vi "syncDAQ_main.vi"() -> ()   [LabVIEW 2013]
uses:
  <vilib>/Utility/error.llb/DialogType.ctl
  <vilib>/DAQmx/read.llb/DAQmx Read (Analog 1D DBL 1Chan NSamp).vi
  <vilib>/DAQmx/read.llb/DAQmx Read (Analog 1D Wfm NChan NSamp).vi
  <vilib>/DAQmx/miscellaneous.llb/DAQmx Fill In Error Info.vi
  <vilib>/ErrorRing/Error Ring.xnode
panel:
  in  "Ratio":dbl=0.3 caption="复位时间比"
  in  "Vx_Max":dbl=3.0 caption="X向最大电压"
  in  "Vy_Max":dbl=3.0 caption="Y向最大电压"
  in  "N_x":i32=512 caption="采样行数"
  in  "N_y":i32=512 caption="每行采样数"
  in  "StopBtn":bool
  in  "每次采集行数":i32=16
  in  "physical channels read":tag="Dev1/ai0" caption="物理通道（读取）"
  in  "physical channels write":tag="Dev1/ao0:1" caption="物理通道（写入）"
  out "number of samples\nper channel":i32=11703 caption="每通道采样数"
  in  "rate":dbl=250000.0 caption="采样速率" format="%#_6f"
  out "data read":waveform(dbl)[](graph) caption="数据输出"
  out "data write":waveform(dbl)[](graph) caption="数据输出"
  in  "采样模式":enum32{"有限采样", "连续采样"}(tab)=enum."连续采样"
  out "Finite Sample Graph":dbl[][](graph)
  out "Continuous sampling graph":dbl[][](graph)
  # "Basic DAQ\nsettings"
  # "Imaging settings"
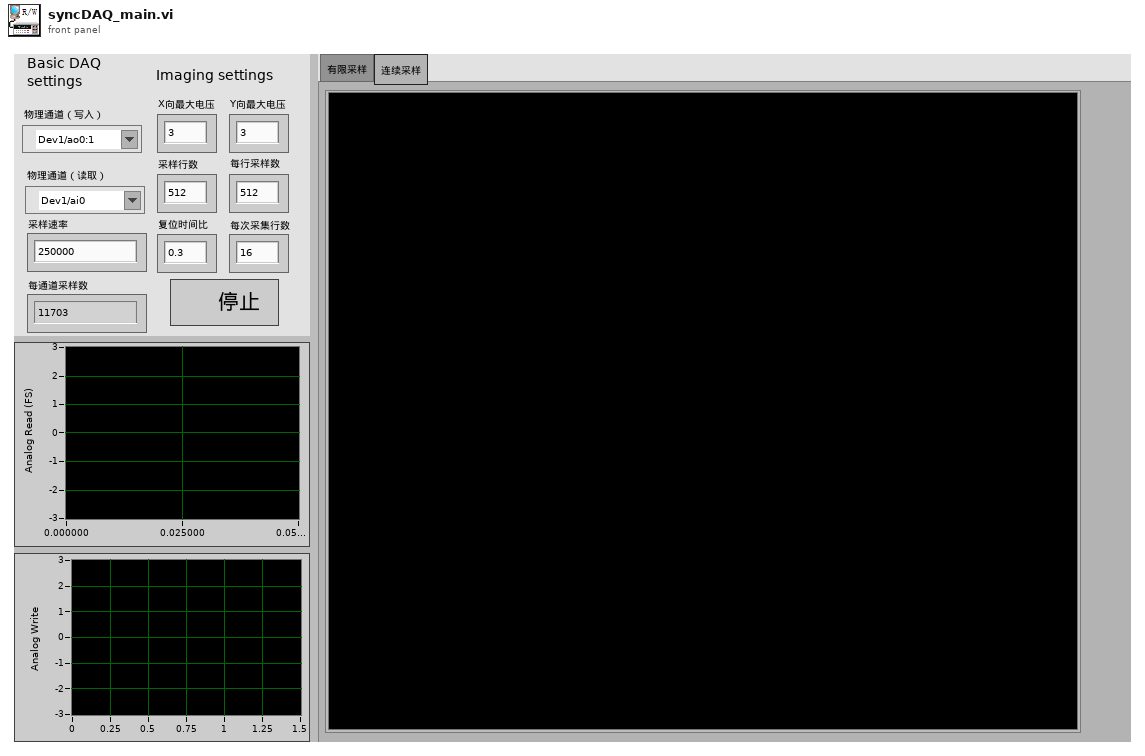
[diagram p1: front panel]
types:
  T1 = enum8{"Enabled", "Disabled", "Disabled and Grayed Out"}
  T2 = cluster{"Vx_Max":dbl, "Vy_Max":dbl, "Tx":dbl, "Row_N":i32, "Ratio":dbl}
  T3 = typedef "DialogType.ctl" = u16
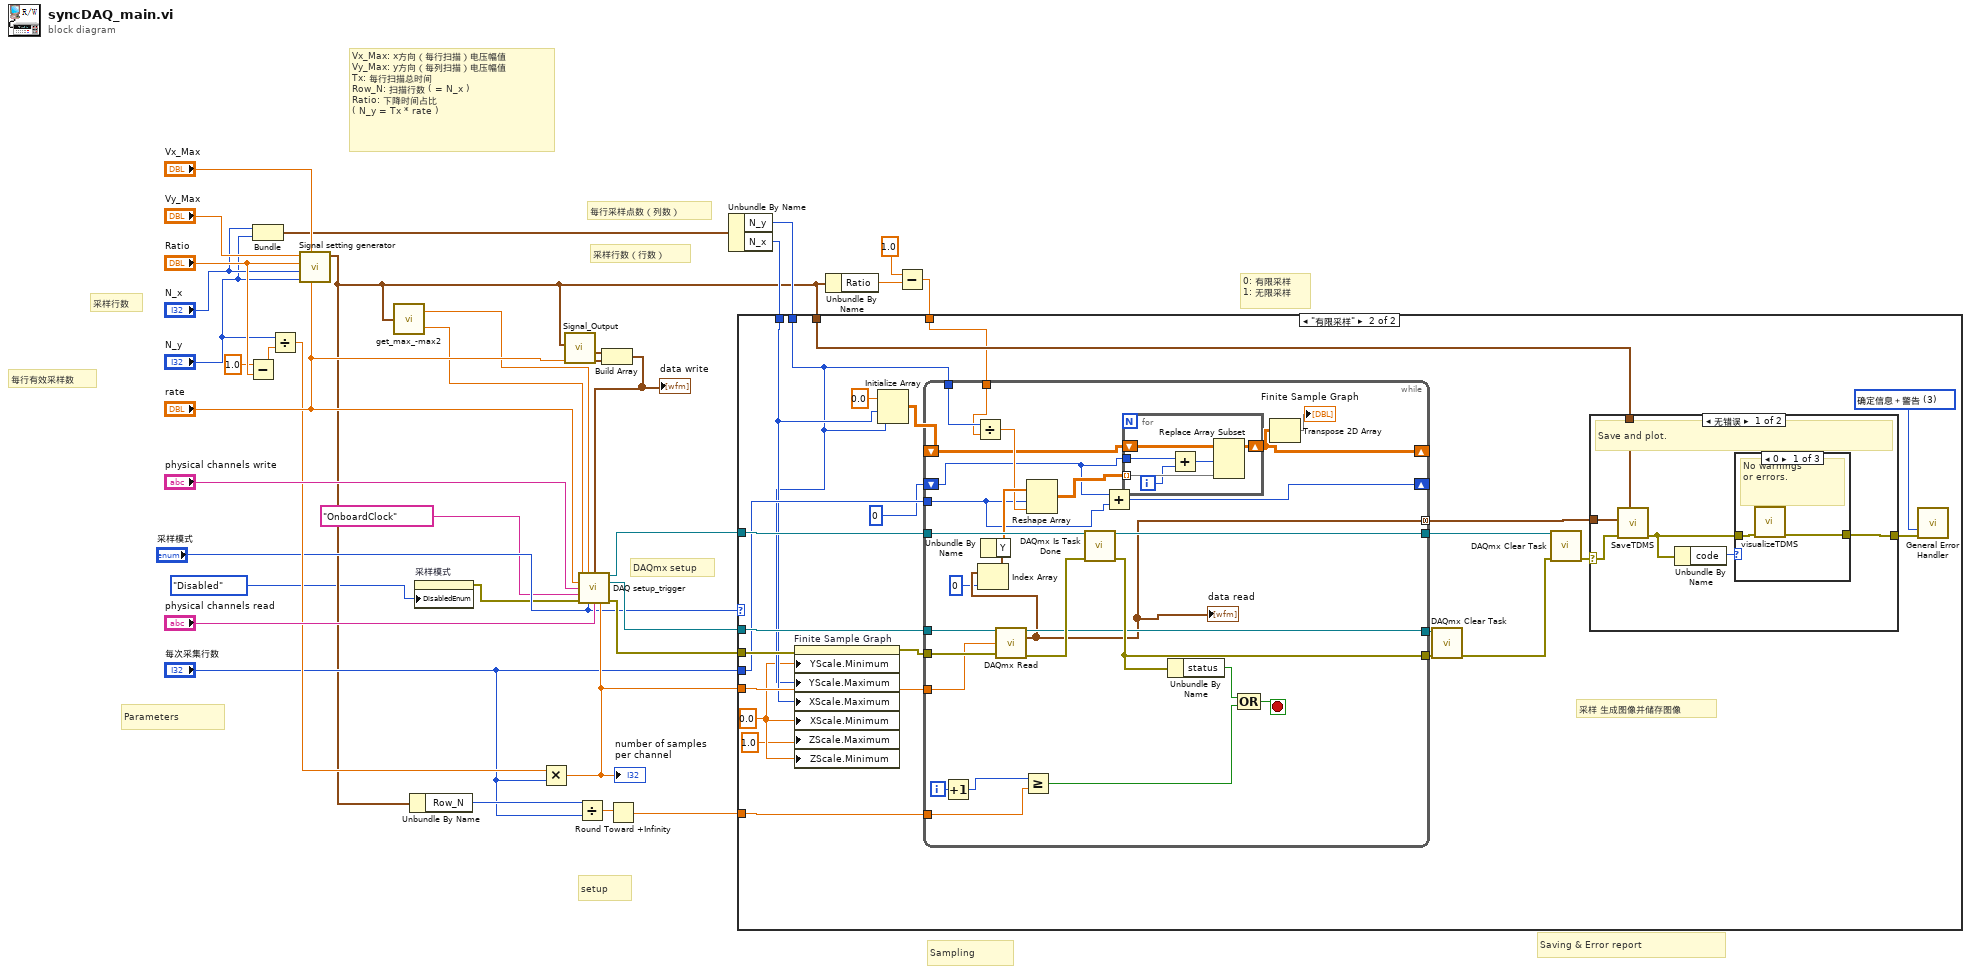
[diagram p0: block diagram]
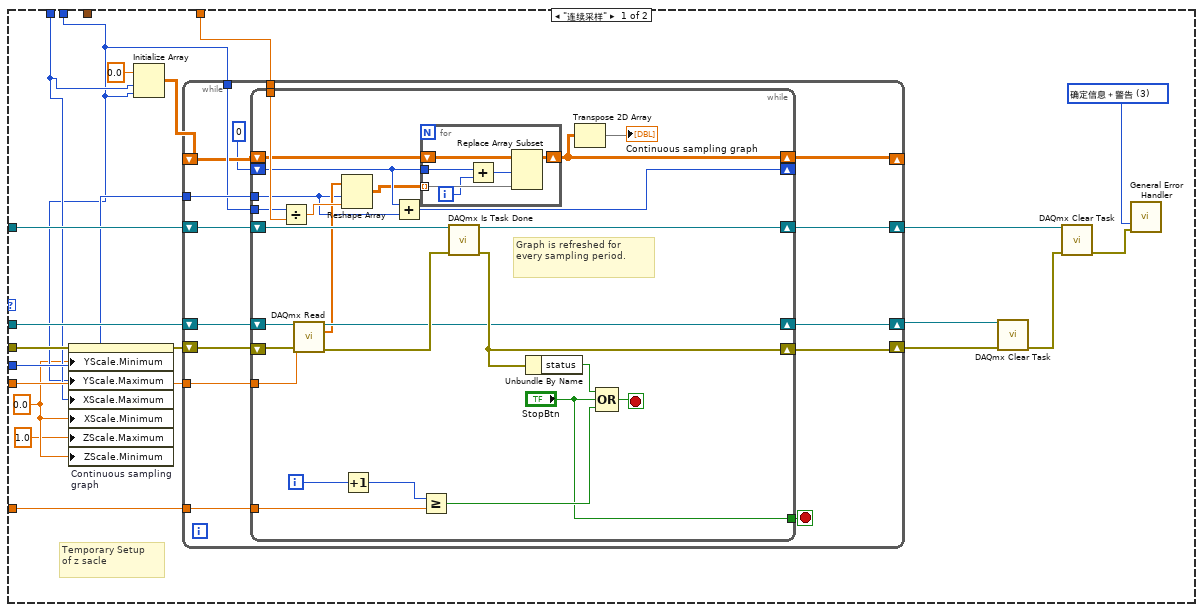
[diagram p2: hidden frame]
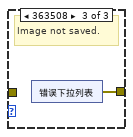
[diagram p4: hidden frame]
diagram:
  # "Vx_Max: x方向（每行扫描）电压幅值\nVy_Max: y方向（每列扫描）电压幅值\nTx: 每行扫描总时间\nRow_N: 扫描行数 ( = N_x )\nRatio: 下降时间占比\n( N_y = Tx * rate )"
  # "采样行数（行数）"
  # "每行采样点数（列数）"
  # "Saving & Error report"
  # "0: 有限采样\n1: 无限采样"
  # "每行有效采样数"
  # "采样行数"
  # "DAQmx setup"
  # "Parameters"
  # "Sampling"
  # "setup"
  n1 = Subtract(x=1.0, y="Ratio") -> (x-y=w22:dbl)
  n2 = Bundle("N_x"="N_x", "N_y"="N_y") -> (w9:cluster{"N_x":i32, "N_y":i32})  [unwired: 1 in]
  n3 = Divide(x="N_y", y=w22) -> (x/y=w21:dbl)
  n4 = call "Signal setting generator.vi"("rate"="rate", "Vx_Max"="Vx_Max", "N_y"="N_y", "N_x"="N_x", "Ratio"="Ratio", "Vy_Max"="Vy_Max") -> ("Waveform out"=w4:T2)  [unwired: 5 in]
  n5 = call "get_max_-max2.vi"("Waveform out"=w4) -> ("-max_xy"=w5:dbl, "max_xy"=w6:dbl)  [unwired: 2 in]
  n6 = Unbundle By Name(w4) -> ("Row_N"=w19:i32)
  n7 = property on="采样模式" class="TabCtl (严格)"("DisabledEnum"=T1."Disabled" ("禁用")) -> (error out=w1:errorcluster)  [unwired: 2 in, 1 out]
  n8 = Multiply(x=w21, y="每次采集行数") -> (x*y=w25:dbl)
  "number of samples\nper channel" <- w25
  n9 = call "Signal_Output.vi"("Fs (Hz)"="rate", "Waveform settings"=w4) -> ("Y"=w29:waveform(dbl), "X"=w30:waveform(dbl))  [unwired: 7 in, 1 out]
  n10 = Divide(x=w19, y="每次采集行数") -> (x/y=w18:dbl)
  n11 = Build Array(w30, w29) -> (w20:waveform(dbl)[])
  "data write" <- w20
  n12 = call "DAQ setup_trigger.vi"("Vx_min"=w5, "Vx_max"=w6, "数组"=w20, "rate"="rate", "physical channels write"="physical channels write", "Timing source"=tag "OnboardClock", "error in"=w1, "sample mode"="采样模式", "physical channels read"="physical channels read", "Number of samples per channel"=w25) -> ("Writing task out"=w35:refnum<k21>, "Reading task out"=w34:refnum<k21>, "错误输出"=w33:errorcluster)  [unwired: 3 in]
  n13 = Round Toward +Infinity(x=w18) -> (ceil(x): smallest int >= x=w17:dbl)
  n14 = Unbundle By Name(w9) -> ("N_y"=w7:i32, "N_x"=w8:i32)
  n15 = Unbundle By Name(w4) -> ("Ratio"=w12:dbl)
  n16 = Subtract(x=1.0, y=w12) -> (x-y=w10:dbl)
  n17 = case shown="\"有限采样\"" "采样模式" {
    tunnel: w35 -> [w55 w126]
    tunnel: w34 -> [w49 w120]
    tunnel: w33 -> [w44 w113]
    tunnel: w25 -> [w48 w117]
    tunnel: w17 -> [w47 w115]
    tunnel: "每次采集行数" -> [w45 w110]
    tunnel: w10 -> [w42 w111]
    tunnel: w8 -> [w40 w106]
    tunnel: w7 -> [w39 w105]
    tunnel: w4 -> [_ w114]
    frame "连续采样" {
      w37 = 0.0 ("X标尺.范围:最小值")
      w50 = T3 3 items=["无对话框", "确定信息", "继续或停止信息", "确定信息＋警告", "继续/停止+警告"] ("type of dialog (OK msg:1)")
      # "Temporary Setup\nof z sacle"
      n18 = property on="Continuous sampling graph" class="IntGraph (严格)"(error in=w44, "YScale.Minimum"=w37, "YScale.Maximum"=w39, "XScale.Maximum"=w40, "XScale.Minimum"=w37, "ZScale.Maximum"=1.0 ("X标尺.范围:最小值"), "ZScale.Minimum"=w37) -> (error out=w43:errorcluster)  [unwired: 1 in, 1 out]
      n19 = Initialize Array(0.0 ("元素"), w40, w39) -> (w38:dbl[][])
      n20 = while {
        tunnel: w48 -> [w66]
        tunnel: w47 -> [w65]
        tunnel: w45 -> [w63]
        tunnel: w42 -> [w62]
        shift-right: [w61] -> w52
        shift-left: w55 -> [w70]
        shift-right: [w69] -> w54
        shift-left: w49 -> [w68]
        shift-right: [w59] -> w53
        shift-left: w43 -> [w67]
        tunnel: w39 -> [w60]
        shift-right: [w57] -> _
        shift-left: w38 -> [w58]
        stop <- w64 stop-if-true
        n21 = while {
          tunnel: w66 -> [w91]
          tunnel: w65 -> [w88]
          shift-right: [w73] -> w57
          shift-left: w58 -> [w74]
          tunnel: ["StopBtn"] -> w64
          tunnel: w63 -> [w75]
          tunnel: w62 -> [w82]
          shift-right: [w81] -> w61
          shift-left: w70 -> [w84]
          shift-right: [w94] -> w69
          shift-left: w68 -> [w92]
          shift-right: [w95] -> w59
          shift-left: w67 -> [w93]
          tunnel: w60 -> [w79]
          shift-right: [w76] -> _
          shift-left: 0 -> [w72]
          i -> [w83]
          stop <- w86 stop-if-true
          # "Graph is refreshed for\nevery sampling period."
          n22 = Divide(x=w79, y=w82) -> (x/y=w80:dbl)
          n23 = call-poly <vilib>:"DAQmx Read.vi"("task/channels in"=w92, "number of samples per channel"=w91, "error in"=w93) -> ("task out"=w94:refnum<k21>, "data"=w77:dbl[], "error out"=w96:errorcluster)  [unwired: 10 in]
          n24 = Reshape Array(w77, w75, w80) -> (w71:dbl[][])
          n25 = Increment(x=w83) -> (x+1=w89:i32)
          n26 = Add(x=w72, y=w75) -> (x+y=w76:i32)
          n27 = for {
            tunnel: w72 -> [w99]
            tunnel: w71 -> [w100] mode=indexing
            shift-right: [w101] -> w73
            shift-left: w74 -> [w102]
            i -> [w98]
            n28 = Add(x=w99, y=w98) -> (x+y=w97:i32)
            n29 = Replace Array Subset(array=w102, new element=w100, index (row)=w97) -> (w101:dbl[][])  [unwired: 1 in]
          }
          n30 = Greater Or Equal?(x=w89, y=w88) -> (x >= y?=w87:bool)
          n31 = call <vilib>:"DAQmx Is Task Done.vi"("task/channels in"=w84, "error in"=w96) -> ("task out"=w81:refnum<k21>, "error out"=w95:errorcluster)  [unwired: 11 in, 1 out]
          n32 = Unbundle By Name(w95) -> ("status"=w90:bool)
          n33 = Transpose 2D Array(2D array=w73) -> (transposed array=→"Continuous sampling graph":dbl[][])
          n34 = Compound Arithmetic op=OR(w90, "StopBtn", w87) -> (w86:bool)
        }
      }
      n35 = call <vilib>:"DAQmx Clear Task.vi"("task in"=w54, "error in"=w53) -> ("error out"=w51:errorcluster)  [unwired: 13 in]
      n36 = call <vilib>:"DAQmx Clear Task.vi"("task in"=w52, "error in"=w51) -> ("error out"=w46:errorcluster)  [unwired: 13 in]
      n37 = call <vilib>:"General Error Handler.vi"("type of dialog (OK msg:1)"=w50, "error in (no error)"=w46) -> ()  [unwired: 9 in, 5 out]
    }
    frame "有限采样" {
      w104 = 0.0 ("X标尺.范围:最小值")
      w121 = T3 3 items=["无对话框", "确定信息", "继续或停止信息", "确定信息＋警告", "继续/停止+警告"] ("type of dialog (OK msg:1)")
      # "采样 生成图像并储存图像"
      n38 = property on="Finite Sample Graph" class="IntGraph (严格)"(error in=w113, "YScale.Minimum"=w104, "YScale.Maximum"=w105, "XScale.Maximum"=w106, "XScale.Minimum"=w104, "ZScale.Maximum"=1.0 ("Z标尺.范围:最小值"), "ZScale.Minimum"=w104) -> (error out=w112:errorcluster)  [unwired: 1 in, 1 out]
      n39 = Initialize Array(0.0 ("元素"), w106, w105) -> (w107:dbl[][])
      n40 = while {
        tunnel: w120 -> [w160]
        tunnel: w126 -> [w163]
        tunnel: w112 -> [w161]
        tunnel: [w165] -> w124
        tunnel: [w164] -> w125
        tunnel: [w162] -> w123
        tunnel: w117 -> [w159]
        tunnel: w115 -> [w154]
        tunnel: [w152] -> w116 mode=concatenating
        shift-right: [w139] -> _
        shift-left: w107 -> [w143]
        tunnel: w111 -> [w148]
        tunnel: w105 -> [w149]
        tunnel: w110 -> [w145]
        shift-right: [w144] -> _
        shift-left: 0 -> [w141]
        i -> [w156]
        stop <- w158 stop-if-true
        n41 = Increment(x=w156) -> (x+1=w155:i32)
        n42 = Divide(x=w149, y=w148) -> (x/y=w146:dbl)
        n43 = call-poly <vilib>:"DAQmx Read.vi"("task/channels in"=w160, "number of samples per channel"=w159, "error in"=w161) -> ("task out"=w164:refnum<k21>, "data"=w152:waveform(dbl)[], "error out"=w166:errorcluster)  [unwired: 10 in]
        "data read" <- w152
        n44 = Index Array(array=w152, index=0 ("索引")) -> (element=w150:waveform(dbl))
        n45 = Unbundle By Name(w150) -> ("Y"=w147:dbl[])
        n46 = Greater Or Equal?(x=w155, y=w154) -> (x >= y?=w153:bool)
        n47 = Reshape Array(w147, w145, w146) -> (w142:dbl[][])
        n48 = call <vilib>:"DAQmx Is Task Done.vi"("task/channels in"=w163, "error in"=w166) -> ("task out"=w162:refnum<k21>, "error out"=w165:errorcluster)  [unwired: 11 in, 1 out]
        n49 = Add(x=w141, y=w145) -> (x+y=w144:i32)
        n50 = for {
          tunnel: w141 -> [w169]
          tunnel: w142 -> [w170] mode=indexing
          shift-right: [w171] -> w139
          shift-left: w143 -> [w172]
          i -> [w168]
          n51 = Add(x=w169, y=w168) -> (x+y=w167:i32)
          n52 = Replace Array Subset(array=w172, new element=w170, index (row)=w167) -> (w171:dbl[][])  [unwired: 1 in]
        }
        n53 = Unbundle By Name(w165) -> ("status"=w157:bool)
        n54 = Compound Arithmetic op=OR(w157, w153) -> (w158:bool)
        n55 = Transpose 2D Array(2D array=w139) -> (transposed array=→"Finite Sample Graph":dbl[][])
      }
      n56 = call <vilib>:"DAQmx Clear Task.vi"("task in"=w125, "error in"=w124) -> ("error out"=w122:errorcluster)  [unwired: 13 in]
      n57 = call <vilib>:"DAQmx Clear Task.vi"("task in"=w123, "error in"=w122) -> ("error out"=w118:errorcluster)  [unwired: 13 in]
      n58 = case "条件结构" shown="无错误" w118 {
        selector: w118 -> [w131 w138]
        tunnel: w116 -> [w132 _]
        tunnel: [w128 w138] -> w119
        tunnel: w114 -> [w127 _]
        frame No Error {
          # "Save and plot."
          n59 = call "SaveTDMS.vi"("Waveform settings"=w127, "错误输入（无错误）"=w131, "数据"=w132) -> ("错误输出"=w130:errorcluster)  [unwired: 8 in]
          n60 = Unbundle By Name(w130) -> ("code"=w129:i32)
          n61 = case "条件结构" shown="0" w129 {
            tunnel: w130 -> [w134 w135 _]
            tunnel: [w133 w135 w136] -> w128
            frame 0 {
              # "No warnings\nor errors."
              n62 = call "visualizeTDMS.vi"("错误输入（无错误）"=w134) -> ("错误输出"=w133:errorcluster)  [unwired: 8 in, 2 out]
            }
            frame Default {
              # "Pass on W/E."
            }
            frame 363508 {
              # "Image not saved."
              n63 = xnode "错误下拉列表"() -> ("错误输出"=w136:errorcluster)
            }
          }
        }
        frame Error {
        }
      }
      n64 = call <vilib>:"General Error Handler.vi"("type of dialog (OK msg:1)"=w121, "error in (no error)"=w119) -> ()  [unwired: 9 in, 5 out]
    }
  }
